vi "Charging _Calc Compensated Temperature.vi"(5 "target temperature (C)":dbl=nan format="%.5f", 6 "error in":errorcluster, 7 "Abort Threshold (42 C)":dbl=42.0 format="%5.5f", 8 "Critical Threshold (41 C)":dbl=41.0 format="%5.5f", 9 "Warning Threshold (40 C)":dbl=40.0 format="%5.5f") -> (0 "error out":errorcluster, 2 "interpolation error":dbl=nan format="%.5f", 3 "compensated temperature (C)":dbl=nan format="%.5f")   [LabVIEW 2010]
uses:
  <vilib>/Analysis/NI_AALPro.lvlib
panel:
  in  "Ideal Thresholds":dbl[](array[numeric])=[40.0, 41.0, 42.0] format="%.5f"
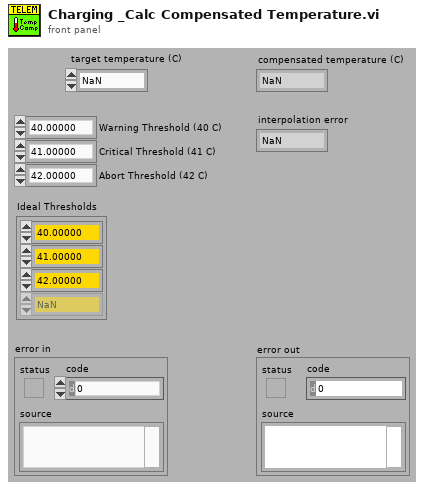
[diagram p1: front panel]
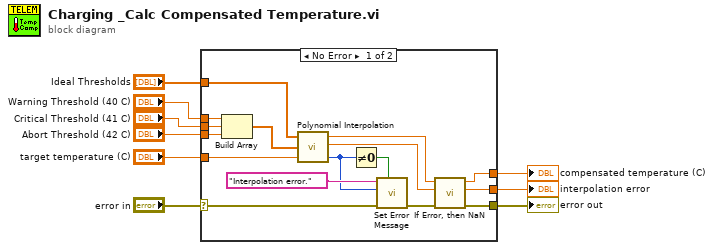
[diagram p0: block diagram]
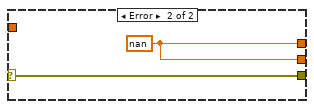
[diagram p2: hidden frame]
diagram:
  n1 = case shown="No Error" "error in" {
    selector: "error in" -> [w19 w27]
    tunnel: "Ideal Thresholds" -> [w25 _]
    tunnel: "target temperature (C)" -> [w24 _]
    tunnel: "Abort Threshold (42 C)" -> [w23 _]
    tunnel: "Critical Threshold (41 C)" -> [w22 _]
    tunnel: "Warning Threshold (40 C)" -> [w21 _]
    tunnel: [w14 w27] -> w3
    tunnel: [w11 w26] -> w2
    tunnel: [w10 w26] -> w1
    frame No Error {
      n2 = Build Array(w21, w22, w23) -> (w20:dbl[])
      n3 = call <vilib>:"Polynomial Interpolation.vi"("x value"=w24, "X"=w20, "Y"=w25) -> ("error"=w16:i32, "interpolation error"=w13:dbl, "interpolation value"=w12:dbl)
      n4 = Not Equal To 0?(x=w16) -> (x != 0?=w18:bool)
      n5 = call "Set Error Message.vi"("enable (T)"=w18, "error in"=w19, "code (-1)"=w16, "message"="Interpolation error." ("Message")) -> ("error out"=w15:errorcluster)  [unwired: 4 in]
      n6 = call "If Error, then NaN.vi"("error in (T)"=w15, "value2"=w13, "value1"=w12) -> ("error out"=w14:errorcluster, "value out2"=w11:dbl, "value out1"=w10:dbl)  [unwired: 3 in, 1 out]
    }
    frame Error {
      w26 = nan ("value out1")
    }
  }
  "compensated temperature (C)" <- w1
  "interpolation error" <- w2
  "error out" <- w3
